vi "CalculateAudioTriggerState.vi"(0 "Low cutoff freq (Hz)":dbl, 1 "element":waveform(dbl), 2 "Audio sample rate (Hz)":i64, 3 "Low buffer in":bool[](array[boolean]), 4 "High Audio Threshold":dbl, 5 "Low Audio Threshold":dbl, 6 "Low monitoring period (s)":dbl, 8 "High cutoff freq (Hz)":dbl, 9 "Samples per\nacquisition chunk":i32, 10 "High buffer in":bool[](array[boolean]), 11 "Low Audio Threshold %":dbl, 12 "High Audio Threshold %":dbl, 14 "High monitoring period (s)":dbl) -> (18 "Mean above high threshold for required %":bool, 20 "Updated high buffer out":bool[](array[boolean]), 21 "Updated low buffer out":bool[](array[boolean]), 22 "Mean under low threshold for required %":bool, 23 "% of period above high threshold":dbl, 24 "% of period below low threshold":dbl, 25 "Filtered audio amplitude":dbl(graph), 26 "Filtered audio":waveform(dbl)(graph))   [LabVIEW 2017]
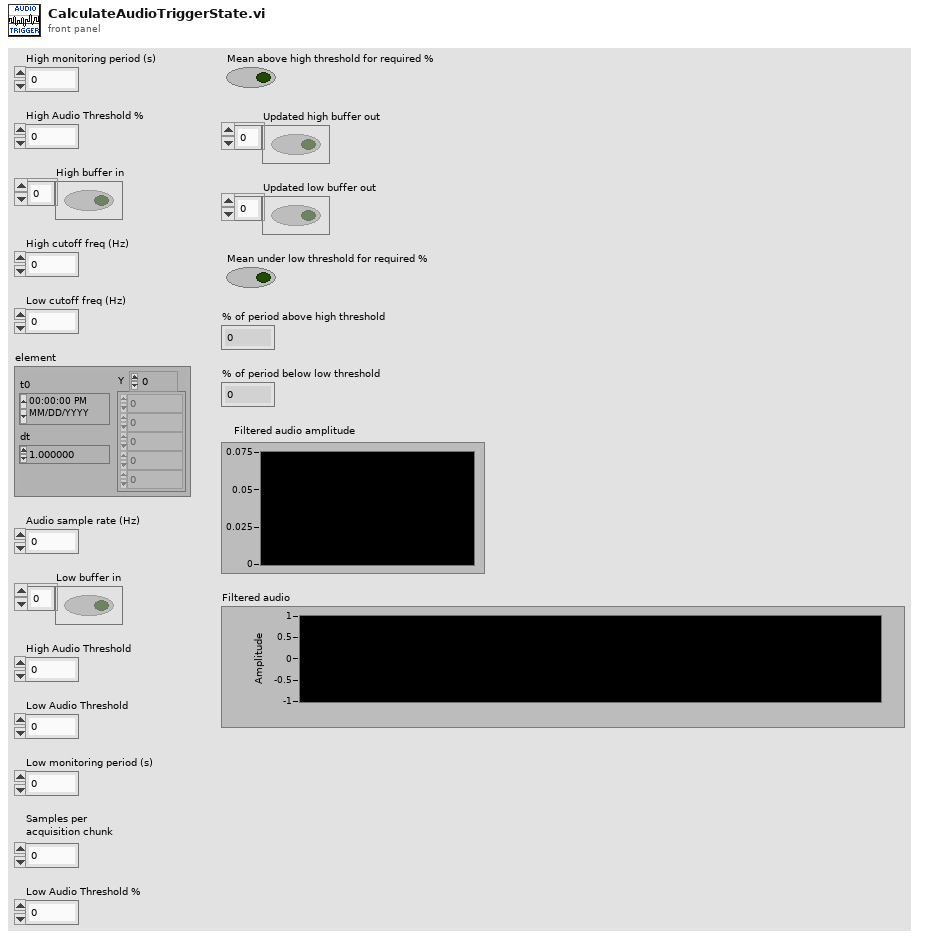
[diagram p1: front panel]
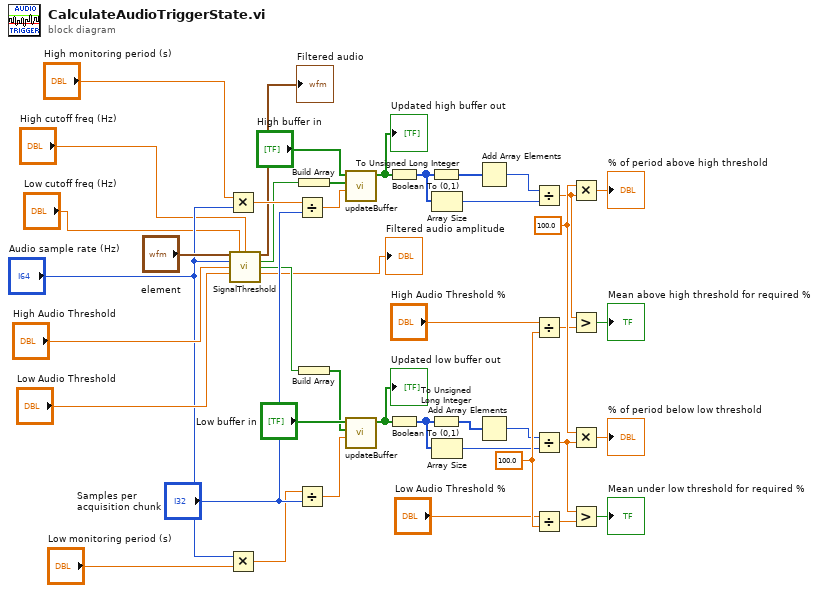
[diagram p0: block diagram]
diagram:
  w35 = 100.0 ("x")
  w30 = 100.0 ("y")
  n1 = Multiply(x="High monitoring period (s)", y="Audio sample rate (Hz)") -> (x*y=w39:dbl)
  n2 = Multiply(x="Audio sample rate (Hz)", y="Low monitoring period (s)") -> (x*y=w10:dbl)
  n3 = call "SignalThreshold.vi"("Signal in"="element", "Low cutoff freq (Hz)"="Low cutoff freq (Hz)", "High cutoff freq (Hz)"="High cutoff freq (Hz)", "Audio sample rate (Hz)"="Audio sample rate (Hz)", "High threshold (Vrms)"="High Audio Threshold", "Low threshold (Vrms)"="Low Audio Threshold") -> ("Filtered signal"=→"Filtered audio":waveform(dbl), "Mean above high threshold?"=w24:bool, "Mean below low threshold?"=w25:bool, "Amplitude"=→"Filtered audio amplitude":dbl)  [unwired: 6 in]
  n4 = Divide(x=w39, y="Samples per\nacquisition chunk") -> (x/y=w38:dbl)
  n5 = Divide(x=w10, y="Samples per\nacquisition chunk") -> (x/y=w40:dbl)
  n6 = Build Array(w24) -> (w9:bool[])
  n7 = Build Array(w25) -> (w11:bool[])
  n8 = call "updateBuffer.vi"("Buffer size"=w38, "New elements"=w9, "Buffer in"="High buffer in") -> ("Updated buffer"=w36:bool[])  [unwired: 8 in]
  "Updated high buffer out" <- w36
  n9 = call "updateBuffer.vi"("Buffer size"=w40, "New elements"=w11, "Buffer in"="Low buffer in") -> ("Updated buffer"=w37:bool[])  [unwired: 8 in]
  "Updated low buffer out" <- w37
  n10 = Boolean To (0,1)(Boolean=w36) -> (0, 1=w13:i16[])
  n11 = Boolean To (0,1)(Boolean=w37) -> (0, 1=w18:i16[])
  n12 = To Unsigned Long Integer(number=w13) -> (unsigned 32bit integer=w43:u32[])
  n13 = To Unsigned Long Integer(number=w18) -> (unsigned 32bit integer=w42:u32[])
  n14 = Array Size(array=w13) -> (size(s)=w14:i32)
  n15 = Array Size(array=w18) -> (size(s)=w17:i32)
  n16 = Add Array Elements(numeric array=w43) -> (sum=w12:u32)
  n17 = Add Array Elements(numeric array=w42) -> (sum=w16:u32)
  n18 = Divide(x=w12, y=w14) -> (x/y=w15:dbl)
  n19 = Divide(x="High Audio Threshold %", y=w30) -> (x/y=w26:dbl)
  n20 = Divide(x=w16, y=w17) -> (x/y=w19:dbl)
  n21 = Divide(x="Low Audio Threshold %", y=w30) -> (x/y=w28:dbl)
  n22 = Multiply(x=w35, y=w15) -> (x*y=→"% of period above high threshold":dbl)
  n23 = Greater?(x=w15, y=w26) -> (0:→"Mean above high threshold for required %":bool)
  n24 = Multiply(x=w35, y=w19) -> (x*y=→"% of period below low threshold":dbl)
  n25 = Greater?(x=w19, y=w28) -> (0:→"Mean under low threshold for required %":bool)
